vi "Wybor rejestratora serial.vi"(6 "Karta":T1, 8 "error in (no error)":errorcluster, 11 "Konfiguracja in":path=path "C:/Users/user/Documents/Rudpol2/Konfiguracja") -> (0 "error out":errorcluster, 2 "znaleziono?":bool, 3 "Plik":string)   [LabVIEW 2014]
uses:
  Kontrolki/KartaDAQ/DAQ card Dane.ctl
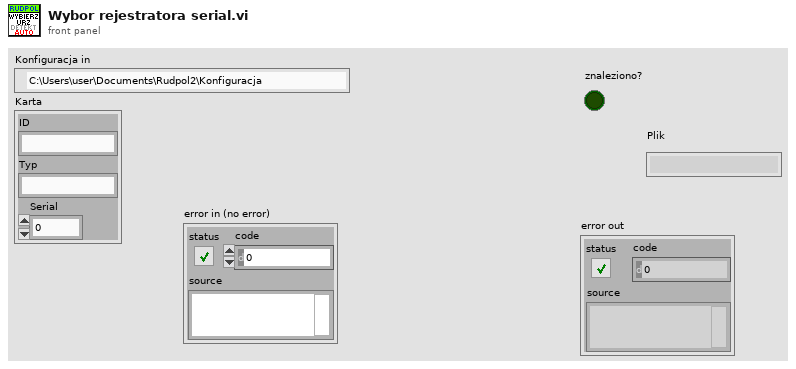
[diagram p1: front panel]
types:
  T1 = typedef "DAQ card Dane.ctl" = cluster{"ID":string, "Typ":string, "Serial":u32}
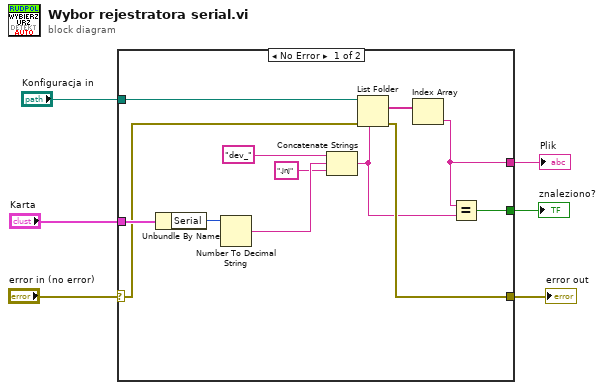
[diagram p0: block diagram]
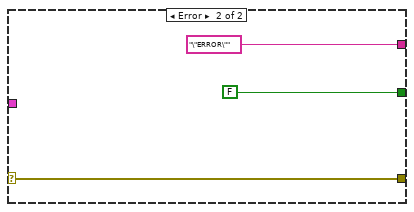
[diagram p2: hidden frame]
diagram:
  n1 = case shown="No Error" "error in (no error)" {
    selector: "error in (no error)" -> [w12 w20]
    tunnel: "Konfiguracja in" -> [w18 _]
    tunnel: [w9 "\"ERROR\""] -> w4
    tunnel: [w10 w20] -> w6
    tunnel: "Karta" -> [w17 _]
    tunnel: [w7 FALSE] -> w1
    frame No Error {
      n2 = Unbundle By Name(w17) -> ("Serial"=w16:u32)
      n3 = Number To Decimal String(number=w16) -> (decimal integer string=w15:string)  [unwired: 1 in]
      n4 = Concatenate Strings("dev_" ("pattern"), w15, ".jnj" ("pattern")) -> (w8:string)
      n5 = List Folder(path=w18, pattern=w8, error in=w12) -> (filenames=w11:string[], error out=w10:errorcluster)  [unwired: 1 in, 2 out]
      n6 = Index Array(array=w11) -> (element=w9:string)  [unwired: 1 in]
      n7 = Equal?(x=w9, y=w8) -> (x = y?=w7:bool)
    }
    frame Error {
    }
  }
  "Plik" <- w4
  "error out" <- w6
  "znaleziono?" <- w1
